vi "New Station Config Item.vi"(10 "Key":string, 11 "Station Config in":T1) -> (3 "Station Config out":T1)   [LabVIEW 2025, in "Full User Interface.lvlib"]
uses:
  Full User Interface.lvlib
  Station Config.ctl
  Station Info.ctl
  Localization/Section.ctl
  Localization/Localization.lvlib
panel:
  in  "Disable":bool caption="禁用"
  in  "Cancel":bool
  in  "OK":bool
  in  "SeqFilename":path caption="序列路径"
  in  "NumberOfSocket":i32=1 caption="总槽位数" min=1 max=255
  out "Station":i32 caption="工站" min=0 step=1
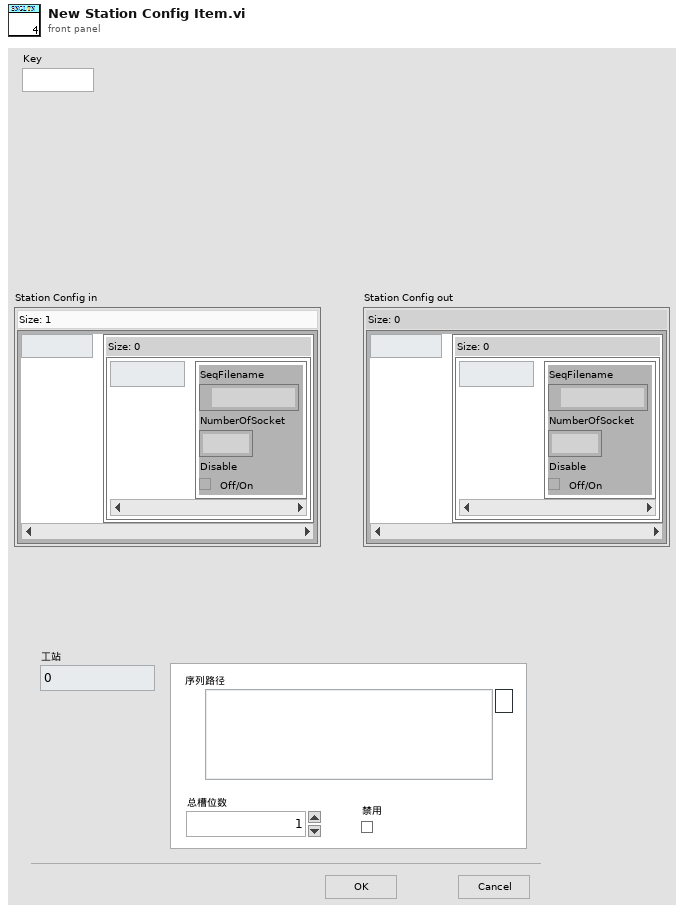
[diagram p1: front panel]
types:
  T1 = typedef "Full User Interface.lvlib/Station Config.ctl" = map{string, map{i32, T2}}
  T2 = typedef "Full User Interface.lvlib/Station Info.ctl" = cluster{"SeqFilename":path, "NumberOfSocket":i32, "Disable":bool}
  T3 = typedef "Localization.lvlib/Section.ctl" = enum16{"Menu", "Title", "Workstation Config"}
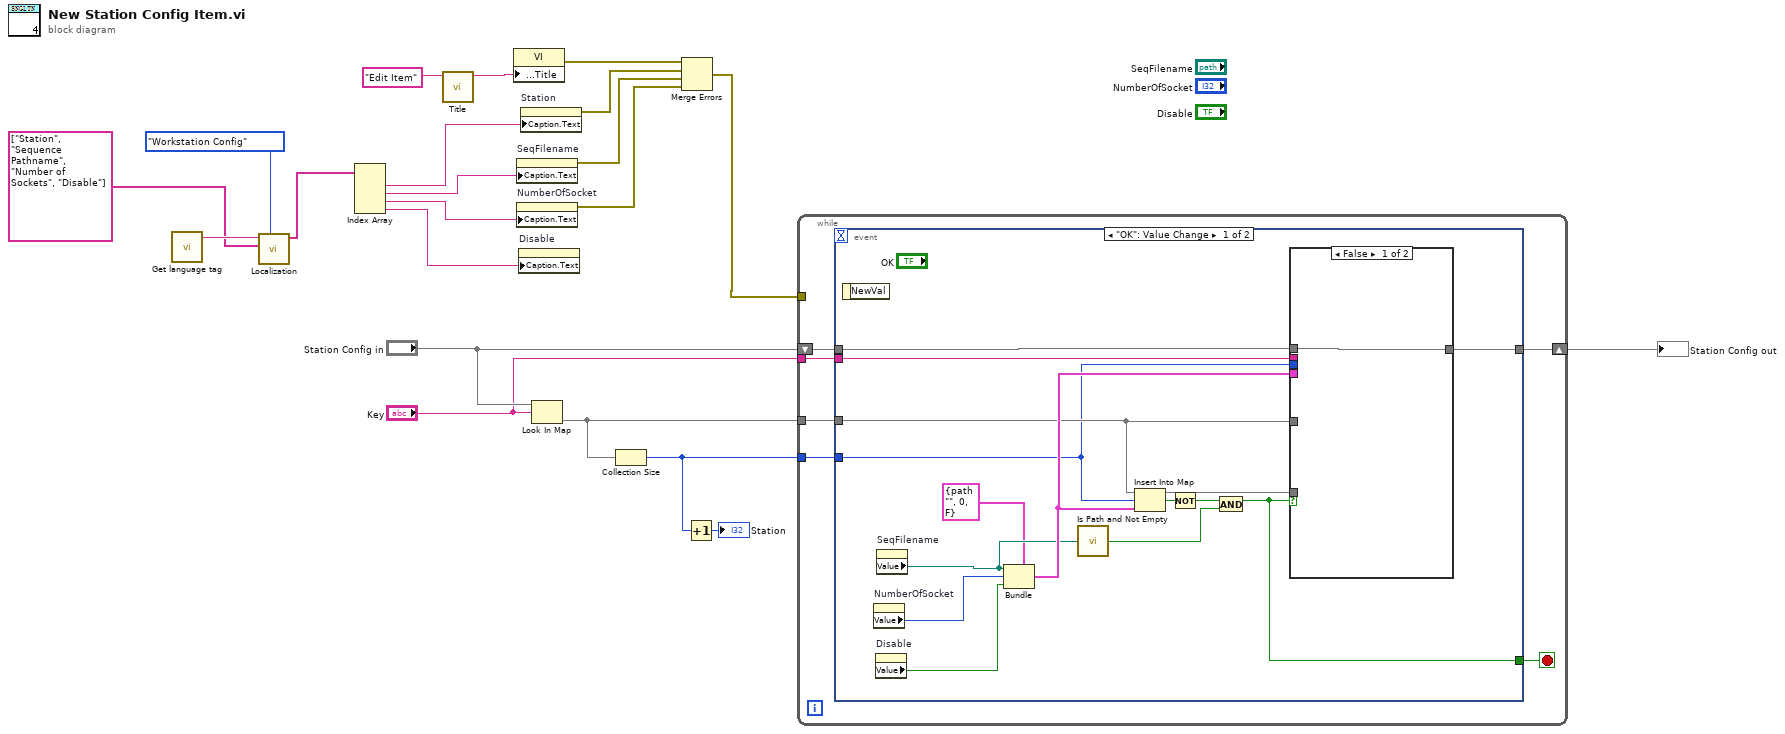
[diagram p0: block diagram]
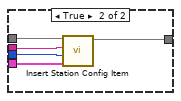
[diagram p2: hidden frame]
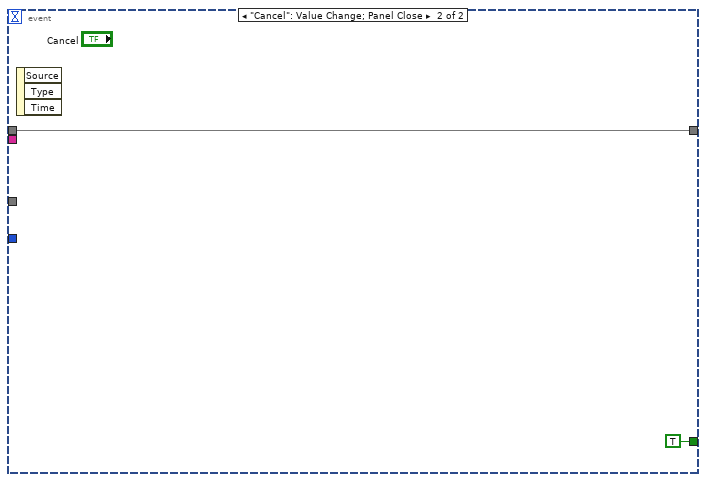
[diagram p3: hidden frame]
diagram:
  n1 = call "Get language tag.vi"() -> ("language tag"=w13:string)  [unwired: 11 in]
  n2 = call "Localization.vi"("section"=Section."Workstation Config", "key"=string[] ["Station", "Sequence Pathname", "Number of Sockets", "Disable"], "Language key"=w13) -> ("Value"=w10:string[])  [unwired: 7 in, 1 out]
  n3 = Index Array(array=w10) -> (element #1=w7:string, element #2=w5:string, element #3=w3:string, element #4=w1:string)  [unwired: 4 in]
  n4 = call "Title.vi"("Front Panel Window:Title"="Edit Item") -> ("Title"=w14:string)  [unwired: 10 in]
  n5 = property on="Property Node" class="VI"("Front Panel.Title"=w14) -> (error out=w9:errorcluster)  [unwired: 2 in, 1 out]
  n6 = property on="SeqFilename" class="Path"("Caption.Text"=w5) -> (error out=w4:errorcluster)  [unwired: 2 in, 1 out]
  n7 = property on="NumberOfSocket" class="DigNum (strict)"("Caption.Text"=w3) -> (error out=w2:errorcluster)  [unwired: 2 in, 1 out]
  n8 = property on="Disable" class="Bool (strict)"("Caption.Text"=w1) -> ()  [unwired: 2 in, 2 out]
  n9 = property on="Station" class="DigNum (strict)"("Caption.Text"=w7) -> (error out=w6:errorcluster)  [unwired: 2 in, 1 out]
  n10 = Look In Map(map="Station Config in", key="Key") -> (value=w18:map{i32, T2})  [unwired: 1 in, 1 out]
  n11 = Collection Size(1:w18) -> (0:w17:i32)
  n12 = Merge Errors(w9, w6, w4, w2) -> (w8:errorcluster)
  n13 = Increment(x=w17) -> (x+1=→"Station":i32)
  n14 = while {
    tunnel: w18 -> [w27]
    tunnel: "Key" -> [w24]
    shift-right: [w25] -> w20
    shift-left: "Station Config in" -> [w26]
    tunnel: w17 -> [w22]
    tunnel: w8 -> [_]
    stop <- w23 stop-if-true
    n15 = event shown="[0] \"OK\": Value Change" {
      selector: _ -> [_ _]
      dyn-events: _ -> [_ _]
      timeout: _ -> [_ _]
      tunnel: w27 -> [w31 _]
      tunnel: w26 -> [w41 w50]
      tunnel: [w40 w50] -> w25
      tunnel: w24 -> [w39 _]
      tunnel: [w33 TRUE] -> w23
      tunnel: w22 -> [w30 _]
      event "OK": Value Change {
        n16 = event-data() -> ()  [unwired: 1 in, 1 out]
        n17 = property on="NumberOfSocket" class="DigNum (strict)"() -> ("Value"=w38:i32)  [unwired: 2 in, 2 out]
        n18 = property on="Disable" class="Bool (strict)"() -> ("Value"=w29:bool)  [unwired: 2 in, 2 out]
        n19 = property on="SeqFilename" class="Path"() -> ("Value"=w35:path)  [unwired: 2 in, 2 out]
        n20 = Bundle(cluster=T2 {"SeqFilename"=path "", "NumberOfSocket"=0, "Disable"=FALSE} ("value"), "SeqFilename"=w35, "NumberOfSocket"=w38, "Disable"=w29) -> (w37:T2)
        n21 = call <vilib>:"Is Path and Not Empty.vi"("path"=w35) -> ("Is Path and Not Empty?"=w32:bool)  [unwired: 4 in]
        n22 = Insert Into Map(map in=w31, key=w30, value=w37) -> (map out=w42:map{i32, T2}, key already included?=w36:bool)  [unwired: 1 out]
        n23 = Not(x=w36) -> (.not. x?=w34:bool)
        n24 = And(x=w34, y=w32) -> (x .and. y?=w33:bool)
        n25 = case shown="False" w33 {
          tunnel: w42 -> [_ _]
          tunnel: w31 -> [_ _]
          tunnel: w41 -> [w43 w48]
          tunnel: [w43 w47] -> w40
          tunnel: w39 -> [_ w46]
          tunnel: w30 -> [_ w45]
          tunnel: w37 -> [_ w44]
          frame False {
          }
          frame True {
            n26 = call "Insert Station Config Item.vi"("value"=w44, "Station"=w45, "Key"=w46, "Station Config in"=w48) -> ("Station Config out"=w47:T1)  [unwired: 7 in]
          }
        }
      }
      event "Cancel": Value Change; Panel Close {
        n27 = event-data() -> ()  [unwired: 1 in, 3 out]
      }
    }
  }
  "Station Config out" <- w20
